vi "Get Basic FP Settings.vi"(8 "error in (no error)":errorcluster, 11 "vi reference":refnum<vi>) -> (0 "error out":errorcluster, 2 "basic fp settings":T1, 3 "vi reference out":refnum<vi>)   [LabVIEW 2020]
uses:
  Basic FP Settings--cluster.ctl
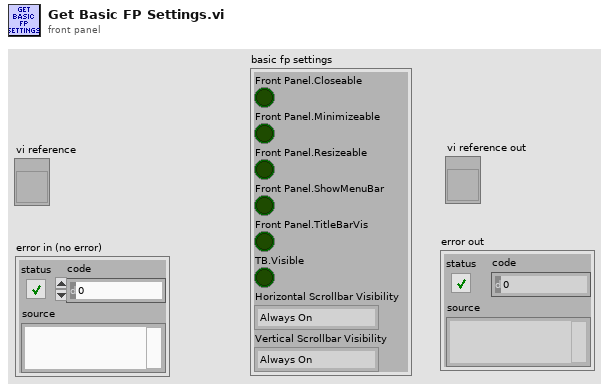
[diagram p1: front panel]
types:
  T1 = typedef "Basic FP Settings--cluster.ctl" = cluster{"Front Panel.Closeable":bool, "Front Panel.Minimizeable":bool, "Front Panel.Resizeable":bool, "Front Panel.ShowMenuBar":bool, "Front Panel.TitleBarVis":bool, "TB.Visible":bool, "Horizontal Scrollbar Visibility":enum16{"Always On", "Always Off", "Off While Running"}, "Vertical Scrollbar Visibility":enum16{"Always On", "Always Off", "Off While Running"}}
  T2 = enum16{"Always On", "Always Off", "Off While Running"}
  T3 = cluster{"Front Panel.Closeable":bool, "Front Panel.Minimizeable":bool, "Front Panel.Resizeable":bool, "Front Panel.ShowMenuBar":bool, "Front Panel.TitleBarVis":bool, "TB.Visible":bool, "HorizScrollbarVisibility":enum16{"Always On", "Always Off", "Off While Running"}, "VertScrollbarVisibility":enum16{"Always On", "Always Off", "Off While Running"}}
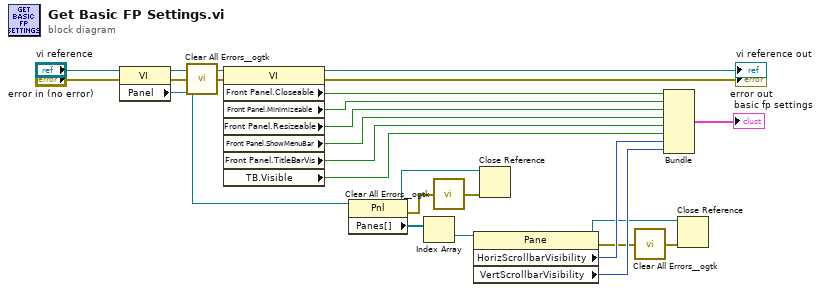
[diagram p0: block diagram]
diagram:
  n1 = property class="VI"(reference="vi reference", error in="error in (no error)") -> (reference out=w11:refnum<vi>, error out=w9:errorcluster, "Panel"=w10:refnum<vi>)
  n2 = call <userlib>:"Clear All Errors__ogtk.vi"("Error In"=w9) -> ("Error Out"=w5:errorcluster)  [unwired: 3 in]
  n3 = property class="VI"(reference=w11, error in=w5) -> (reference out=→"vi reference out":refnum<vi>, error out=→"error out":errorcluster, "Front Panel.Closeable"=w25:bool, "Front Panel.Minimizeable"=w24:bool, "Front Panel.Resizeable"=w23:bool, "Front Panel.ShowMenuBar"=w22:bool, "Front Panel.TitleBarVis"=w21:bool, "TB.Visible"=w20:bool)
  n4 = property class="Pnl"(reference=w10) -> (reference out=w4:refnum<vi>, error out=w7:errorcluster, "Panes[]"=w16:refnum<vi>[])  [unwired: 1 in]
  n5 = Index Array(array=w16) -> (element=w15:refnum<vi>)  [unwired: 1 in]
  n6 = call <userlib>:"Clear All Errors__ogtk.vi"("Error In"=w7) -> ("Error Out"=w3:errorcluster)  [unwired: 3 in]
  n7 = property class="Pane"(reference=w15) -> (reference out=w1:refnum<vi>, error out=w6:errorcluster, "HorizScrollbarVisibility"=w14:T2, "VertScrollbarVisibility"=w13:T2)  [unwired: 1 in]
  n8 = Close Reference(reference=w4, error in (no error)=w3) -> ()  [unwired: 1 out]
  n9 = call <userlib>:"Clear All Errors__ogtk.vi"("Error In"=w6) -> ("Error Out"=w2:errorcluster)  [unwired: 3 in]
  n10 = Bundle("Front Panel.Closeable"=w25, "Front Panel.Minimizeable"=w24, "Front Panel.Resizeable"=w23, "Front Panel.ShowMenuBar"=w22, "Front Panel.TitleBarVis"=w21, "TB.Visible"=w20, "HorizScrollbarVisibility"=w14, "VertScrollbarVisibility"=w13) -> (→"basic fp settings":T3)  [unwired: 1 in]
  n11 = Close Reference(reference=w1, error in (no error)=w2) -> ()  [unwired: 1 out]
